vi "daqtestv2.vi"() -> ()   [LabVIEW 2015]
uses:
  <vilib>/Waveform/WDTOps.llb/WDT Append Waveforms DBL.vi
  <vilib>/Waveform/WDTFileIO.llb/Export Waveform To Spreadsheet File.vi
panel:
  out "Waveform Chart 2":dynamicdata(graph)
  in  "stop":bool
  out "Waveform Chart":waveform(dbl)(graph)
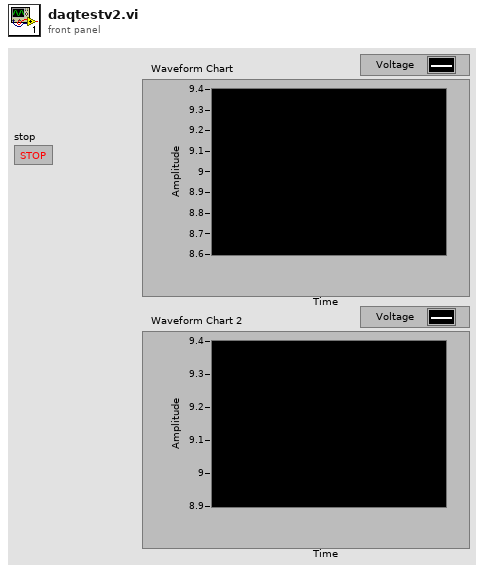
[diagram p1: front panel]
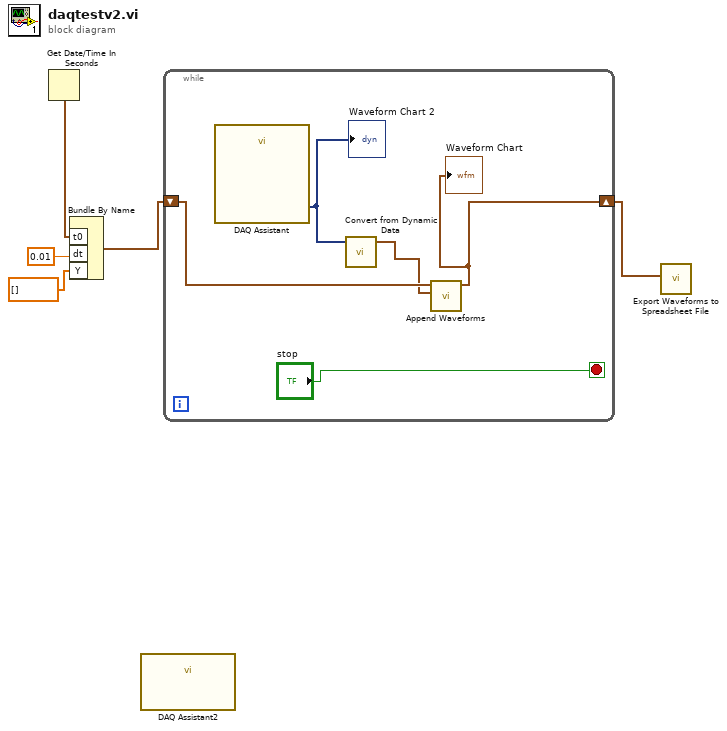
[diagram p0: block diagram]
diagram:
  n1 = Get Date/Time In Seconds() -> (seconds since 1Jan1904=w3:timestamp)
  n2 = Bundle By Name("t0"=w3, "dt"=0.01, "Y"=dbl[] []) -> (w2:waveform(dbl))  [unwired: 1 in]
  n3 = call "DAQ Assistant2"() -> ()  [unwired: 12 in]
  n4 = while {
    shift-right: [w8] -> w1
    shift-left: w2 -> [w10]
    stop <- "stop" stop-if-true
    n5 = call "DAQ Assistant"() -> ("data"=w6:dynamicdata)  [unwired: 17 in, 2 out]
    "Waveform Chart 2" <- w6
    n6 = call "Convert from Dynamic Data"("Dynamic Data Type"=w6) -> ("Waveform"=w9:waveform(dbl))  [unwired: 3 in]
    n7 = call-poly <vilib>:"Append Waveforms.vi"("waveform B"=w9, "waveform A"=w10) -> ("waveform out"=w8:waveform(dbl))  [unwired: 8 in, 1 out]
    "Waveform Chart" <- w8
  }
  n8 = call-poly <vilib>:"Export Waveforms to Spreadsheet File.vi"("waveform"=w1) -> ()  [unwired: 9 in, 2 out]
